vi "Auto_STM.vi"() -> ()   [LabVIEW 2013]
panel:
  out "Output Data":string[](array[string])
  in  "error in (no error)":errorcluster
  in  "Channel List":string
  out "error out":errorcluster
  out "VISA session":refnum<visa-resource-name>
  in  "VISA resource name":refnum<visa-resource-name>
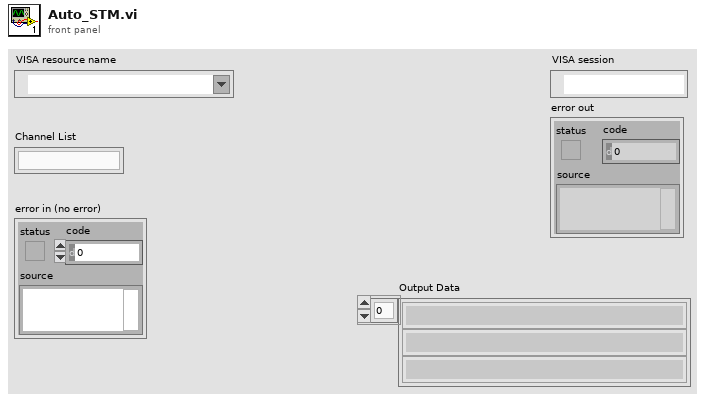
[diagram p1: front panel]
types:
  T1 = enum16{"4 1/2", "5 1/2", "6 1/2", "Least", "Highest", "Default"}
  T2 = enum16{"100 Ohm", "1 kOhm", "10 kOhm", "100 kOhm", "1 MOhm", "10 MOhm", "100 MOhm", "Auto", "Minimum", "Maximum", "Default"}
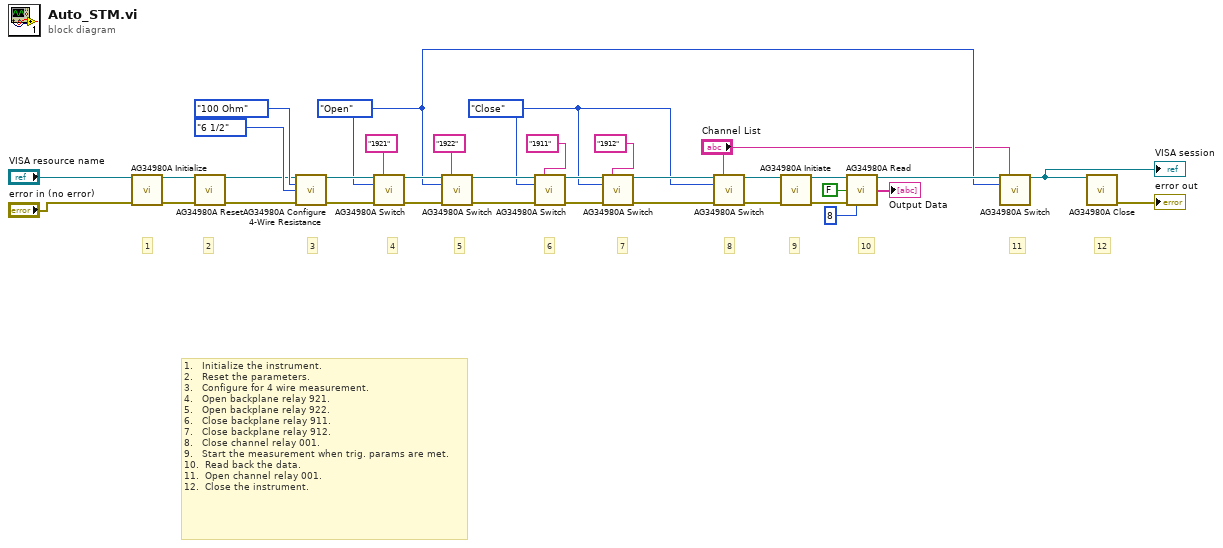
[diagram p0: block diagram]
diagram:
  w14 = enum16{"Close", "Open"}."Close" ("Open/Close (0:Close)")
  w6 = enum16{"Close", "Open"}."Open" ("Open/Close (0:Close)")
  # "1.   Initialize the instrument.\n2.   Reset the parameters.\n3.   Configure for 4 wire measurement.\n4.   Open backplane relay 921.\n5.   Open backplane relay 922.\n6.   Close backplane relay 911.\n7.   Close backplane relay 912.\n8.   Close channel relay 001.\n9.   Start the measurement when trig. params are met.\n10.  Read back the data.\n11.  Open channel relay 001.\n12.  Close the instrument."
  # "12"
  # "11"
  # "10"
  # "9"
  # "8"
  # "7"
  # "6"
  # "5"
  # "4"
  # "3"
  # "2"
  # "1"
  n1 = call <instrlib>:"AG34980A Initialize.vi"("VISA resource name"="VISA resource name", "error in (no error)"="error in (no error)") -> ("VISA session"=w31:refnum<visa-resource-name>, "error out"=w32:errorcluster)  [unwired: 12 in]
  n2 = call <instrlib>:"AG34980A Reset.vi"("VISA resource name"=w31, "error in (no error)"=w32) -> ("VISA resource name out"=w29:refnum<visa-resource-name>, "error out"=w30:errorcluster)  [unwired: 12 in]
  n3 = call <instrlib>:"AG34980A Configure 4-Wire Resistance.vi"("VISA resource name"=w29, "Range (7:Auto)"=T2."100 Ohm", "Resolution (5:Default)"=T1."6 1/2", "error in (no error)"=w30) -> ("VISA resource name out"=w27:refnum<visa-resource-name>, "error out"=w28:errorcluster)  [unwired: 10 in]
  n4 = call <instrlib>:"AG34980A Switch.vi"("VISA resource name"=w27, "Channel List"="1921", "Open/Close (0:Close)"=w6, "error in (no error)"=w28) -> ("VISA resource name out"=w23:refnum<visa-resource-name>, "error out"=w24:errorcluster)  [unwired: 9 in, 1 out]
  n5 = call <instrlib>:"AG34980A Switch.vi"("VISA resource name"=w23, "Channel List"="1922", "Open/Close (0:Close)"=w6, "error in (no error)"=w24) -> ("VISA resource name out"=w20:refnum<visa-resource-name>, "error out"=w19:errorcluster)  [unwired: 9 in, 1 out]
  n6 = call <instrlib>:"AG34980A Switch.vi"("VISA resource name"=w20, "Channel List"="1911", "Open/Close (0:Close)"=w14, "error in (no error)"=w19) -> ("VISA resource name out"=w22:refnum<visa-resource-name>, "error out"=w21:errorcluster)  [unwired: 9 in, 1 out]
  n7 = call <instrlib>:"AG34980A Switch.vi"("VISA resource name"=w22, "Channel List"="1912", "Open/Close (0:Close)"=w14, "error in (no error)"=w21) -> ("VISA resource name out"=w15:refnum<visa-resource-name>, "error out"=w16:errorcluster)  [unwired: 9 in, 1 out]
  n8 = call <instrlib>:"AG34980A Switch.vi"("VISA resource name"=w15, "Channel List"="Channel List", "Open/Close (0:Close)"=w14, "error in (no error)"=w16) -> ("VISA resource name out"=w12:refnum<visa-resource-name>, "error out"=w11:errorcluster)  [unwired: 9 in, 1 out]
  n9 = call <instrlib>:"AG34980A Initiate.vi"("VISA resource name"=w12, "error in (no error)"=w11) -> ("VISA resource name out"=w10:refnum<visa-resource-name>, "error out"=w9:errorcluster)  [unwired: 12 in]
  n10 = call <instrlib>:"AG34980A Read.vi"("VISA resource name"=w10, "Numbers Only (T:On)"=FALSE, "error in (no error)"=w9, "Byte Count (1024 bytes)"=8) -> ("VISA resource name out"=w7:refnum<visa-resource-name>, "Output Data"=→"Output Data":string[])  [unwired: 8 in, 2 out]
  n11 = call <instrlib>:"AG34980A Switch.vi"("VISA resource name"=w7, "Channel List"="Channel List", "Open/Close (0:Close)"=w6) -> ("VISA resource name out"=w3:refnum<visa-resource-name>)  [unwired: 10 in, 2 out]
  "VISA session" <- w3
  n12 = call <instrlib>:"AG34980A Close.vi"("VISA resource name"=w3) -> ("error out"=→"error out":errorcluster)  [unwired: 14 in]
